vi "Process Path.vi"(10 "Lookahead":dbl, 11 "Odometry":T1) -> (1 "Finished?":bool, 2 "Close Point":T2, 3 "Target Point":T2, 5 "index out":i32)   [LabVIEW 2017, in "Pure Pursuit.lvlib"]
uses:
  Pure Pursuit.lvlib
  Typedef/Path Point.ctl
  Odometry/Typedef/Odometry.ctl
  Typedef/Path AE Action.ctl
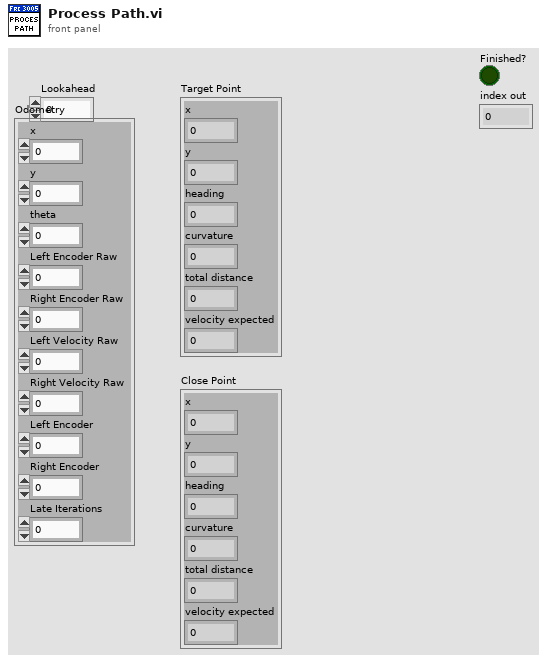
[diagram p1: front panel]
types:
  T1 = typedef "Odometry.ctl" = cluster{"x":dbl, "y":dbl, "theta":dbl, "Left Encoder Raw":i32, "Right Encoder Raw":i32, "Left Velocity Raw":i32, "Right Velocity Raw":i32, "Left Encoder":dbl, "Right Encoder":dbl, "Late Iterations":i16}
  T2 = typedef "Pure Pursuit.lvlib/Path Point.ctl" = cluster{"x":dbl, "y":dbl, "heading":dbl, "curvature":dbl, "total distance":dbl, "velocity expected":dbl}
  T3 = typedef "Pure Pursuit.lvlib/Path AE Action.ctl" = enum16{"Initialize", "Get Close Point", "Get Target Point", "Default", "Get Point", "Get Distance Remaining"}
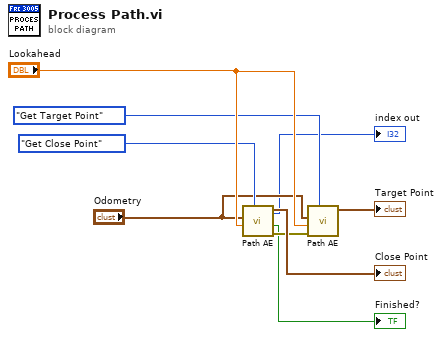
[diagram p0: block diagram]
diagram:
  n1 = call "Path AE.vi"("Path AE Action"=Path_AE_Action."Get Close Point", "Lookahead"="Lookahead", "Odometry"="Odometry") -> ("error out"=w6:errorcluster, "Finished?"=→"Finished?":bool, "point"=→"Close Point":T2, "index out"=→"index out":i32)  [unwired: 3 in, 2 out]
  n2 = call "Path AE.vi"("Path AE Action"=Path_AE_Action."Get Target Point", "error in (no error)"=w6, "Lookahead"="Lookahead", "Odometry"="Odometry") -> ("point"=→"Target Point":T2)  [unwired: 2 in, 5 out]
